vi "Create Instrument Addon Custom Device Node.vi"(8 "Error In":errorcluster, 11 "Target In":refnum<k24>) -> (0 "Error Out":errorcluster, 2 "Instrument Addon Refnum Out":u64, 3 "Target Out":refnum<k24>)   [LabVIEW 2018, in "Instrument Addon Scripting API.lvlib"]
uses:
  Instrument Addon Scripting API.lvlib
  NationalInstruments.VeriStand.SystemDefinitionAPI
  Addon/Addon Shared/SubVIs/Constants.vi
  Addon/Addon Shared/Instrument Addon Shared.lvlib
  <vilib>/NI Veristand/Custom Device Tools/Custom Device Utility Library/Custom Device Utility Library.lvlib
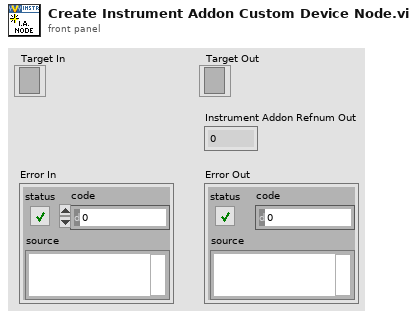
[diagram p1: front panel]
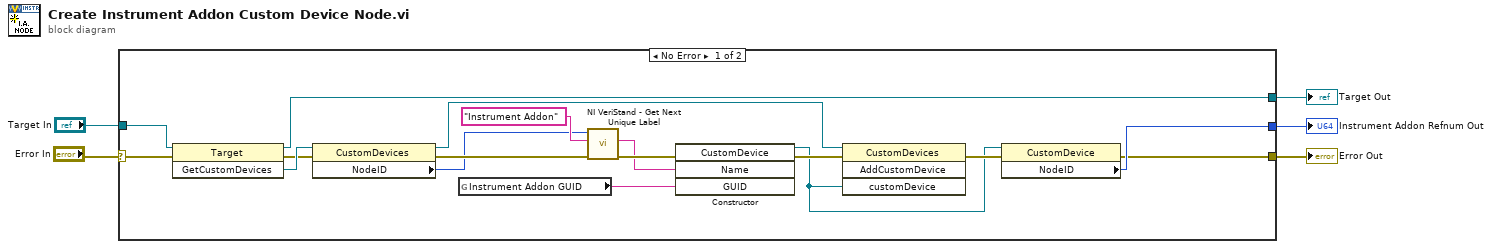
[diagram p0: block diagram]
diagram:
  n1 = case shown="No Error" "Error In" {
    selector: "Error In" -> [w6 w24]
    tunnel: [w22 w23] -> w5
    tunnel: [w21 _] -> w4
    tunnel: [w20 w24] -> w3
    tunnel: "Target In" -> [w18 w23]
    frame No Error {
      n2 = invoke class="Target" method="GetCustomDevices"(reference=w18, error in=w6) -> (reference out=w22:refnum<k24>, error out=w11:errorcluster, "GetCustomDevices"=w19:refnum<k24>)  [unwired: 1 in]
      n3 = property class="CustomDevices"(reference=w19, error in=w11) -> (reference out=w14:refnum<k24>, error out=w16:errorcluster, "NodeID"=w12:u64)
      n4 = global read "Constants.vi" "Instrument Addon GUID"() -> (w10:string)
      n5 = call <vilib>:"NI VeriStand - Get Next Unique Label.vi"("error in (no error)"=w16, "Label"="Instrument Addon" ("Name"), "Parent Ref in"=w12) -> ("error out"=w17:errorcluster, "Label out"=w15:string)  [unwired: 5 in, 2 out]
      n6 = constructor class="CustomDevice"(error in=w17, "Name"=w15, "GUID"=w10) -> (reference out=w7:refnum<k24>, error out=w9:errorcluster)  [unwired: 2 in, 3 out]
      n7 = invoke class="CustomDevices" method="AddCustomDevice"(reference=w14, error in=w9, "customDevice"=w7) -> (error out=w8:errorcluster)  [unwired: 1 in, 3 out]
      n8 = property class="CustomDevice"(reference=w7, error in=w8) -> (error out=w20:errorcluster, "NodeID"=w21:u64)  [unwired: 1 out]
    }
    frame Error {
    }
  }
  "Target Out" <- w5
  "Instrument Addon Refnum Out" <- w4
  "Error Out" <- w3
